vi "SetControlValue.vi"(10 "Value":variant, 11 "ControlVariant":variant) -> (0 "IsControl":bool)   [LabVIEW 2017]
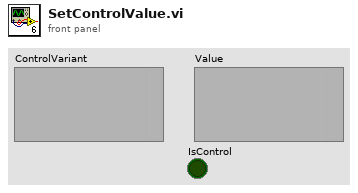
[diagram p1: front panel]
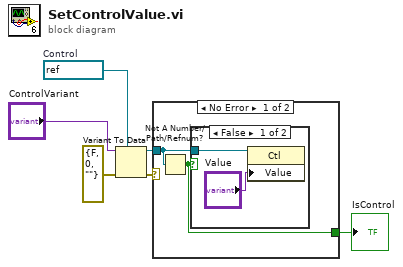
[diagram p0: block diagram]
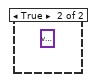
[diagram p2: hidden frame]
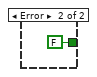
[diagram p3: hidden frame]
diagram:
  w4 = refnum<vi> refnum  # Control
  n1 = Variant To Data(error in=errorcluster {"status"=FALSE, "code"=0, "source"=""}, type=w4, Variant="ControlVariant") -> (data=w6:refnum<vi>, error out=w1:errorcluster)
  n2 = case shown="No Error" w1 {
    tunnel: w6 -> [w8 _]
    tunnel: [w7 FALSE] -> w5
    frame No Error {
      n3 = Not A Number/Path/Refnum?(number/path/refnum=w8) -> (NaN/Path/Refnum?=w7:bool)
      n4 = case shown="False" w7 {
        tunnel: w8 -> [w10 _]
        frame False {
          n5 = property class="Ctl"(reference=w10, "Value"="Value") -> ()  [unwired: 1 in, 2 out]
        }
        frame True {
          (unwired) variant ("Value")
        }
      }
    }
    frame Error {
    }
  }
  "IsControl" <- w5
